vi "TEST Performance Benchmark.vi"() -> ()   [LabVIEW 2011]
panel:
  in  "stop":bool
  in  "source?":bool=TRUE
  in  "Reset Best Time":bool
  out "Best Round Trip Time (ms)":u32
  in  "Parse":bool=TRUE
  in  "Generate":bool=TRUE
  out "Round Trip Time (ms)":u32
  out "Data Round Trip Success?":bool
  in  "Cluster":T1={"Array"=[{"Array"=[{"Array"=[{"Boolean"=FALSE, "Numeric"=0.0, "Numeric 2"=0.0, "Numeric 3"=0.0, "Numeric 4"=0.0}, {"Boolean"=FALSE, "Numeric"=0.0, "Numeric 2"=0.0, "Numeric 3"=0.0, "Numeric 4"=0.0}, {"Boolean"=FALSE, "Numeric"=0.0, "Numeric 2"=0.0, "Numeric 3"=0.0, "Numeric 4"=1.0}], "Numeric"=0.0, "Numeric 2"=0.0, "Numeric 3"=0.0, "Numeric 4"=0.0}, {"Array"=[{"Boolean"=FALSE, "Numeric"=0.0, "Numeric 2"=0.0, "Numeric 3"=0.0, "Numeric 4"=0.0}, {"Boolean"=FALSE, "Numeric"=0.0, "Numeric 2"=0.0, "Numeric 3"=0.0, "Numeric 4"=0.0}, {"Boolean"=FALSE, "Numeric"=0.0, "Numeric 2"=1.0, "Numeric 3"=0.0, "Numeric 4"=0.0}], "Numeric"=0.0, "Numeric 2"=0.0, "Numeric 3"=0.0, "Numeric 4"=0.0}, {"Array"=[{"Boolean"=FALSE, "Numeric"=0.0, "Numeric 2"=0.0, "Numeric 3"=0.0, "Numeric 4"=1.0}, {"Boolean"=FALSE, "Numeric"=0.0, "Numeric 2"=0.0, "Numeric 3"=0.0, "Numeric 4"=0.0}, {"Boolean"=FALSE, "Numeric"=0.0, "Numeric 2"=0.0, "Numeric 3"=0.0, "Numeric 4"=1.0}], "Numeric"=0.0, "Numeric 2"=0.0, "Numeric 3"=0.0, "Numeric 4"=0.0}], "Cluster 2"={"Boolean"=FALSE, "Numeric"=0.0, "Numeric 2"=0.0, "Numeric 3"=0.0, "Numeric 4"=0.0}}, {"Array"=[], "Cluster 2"={"Boolean"=FALSE, "Numeric"=0.0, "Numeric 2"=0.0, "Numeric 3"=0.0, "Numeric 4"=0.0}}, {"Array"=[], "Cluster 2"={"Boolean"=FALSE, "Numeric"=0.0, "Numeric 2"=0.0, "Numeric 3"=0.0, "Numeric 4"=0.0}}, {"Array"=[{"Array"=[{"Boolean"=FALSE, "Numeric"=0.0, "Numeric 2"=0.0, "Numeric 3"=0.0, "Numeric 4"=0.0}, {"Boolean"=FALSE, "Numeric"=0.0, "Numeric 2"=0.0, "Numeric 3"=0.0, "Numeric 4"=0.0}, {"Boolean"=FALSE, "Numeric"=0.0, "Numeric 2"=0.0, "Numeric 3"=0.0, "Numeric 4"=1.0}], "Numeric"=0.0, "Numeric 2"=0.0, "Numeric 3"=0.0, "Numeric 4"=0.0}, {"Array"=[{"Boolean"=FALSE, "Numeric"=0.0, "Numeric 2"=0.0, "Numeric 3"=0.0, "Numeric 4"=0.0}, {"Boolean"=FALSE, "Numeric"=0.0, "Numeric 2"=0.0, "Numeric 3"=0.0, "Numeric 4"=0.0}, {"Boolean"=FALSE, "Numeric"=0.0, "Numeric 2"=0.0, "Numeric 3"=0.0, "Numeric 4"=1.0}], "Numeric"=0.0, "Numeric 2"=0.0, "Numeric 3"=0.0, "Numeric 4"=0.0}, {"Array"=[{"Boolean"=FALSE, "Numeric"=0.0, "Numeric 2"=0.0, "Numeric 3"=0.0, "Numeric 4"=0.0}, {"Boolean"=FALSE, "Numeric"=0.0, "Numeric 2"=0.0, "Numeric 3"=0.0, "Numeric 4"=0.0}, {"Boolean"=FALSE, "Numeric"=0.0, "Numeric 2"=0.0, "Numeric 3"=0.0, "Numeric 4"=1.0}], "Numeric"=0.0, "Numeric 2"=0.0, "Numeric 3"=0.0, "Numeric 4"=1.0}], "Cluster 2"={"Boolean"=FALSE, "Numeric"=0.0, "Numeric 2"=0.0, "Numeric 3"=0.0, "Numeric 4"=0.0}}], "Cluster 2"={"Boolean"=FALSE, "Numeric"=0.0, "Numeric 2"=0.0, "Numeric 3"=0.0, "Numeric 4"=0.0}, "Cluster 3"={"Boolean"=FALSE, "Numeric"=0.0, "Numeric 2"=0.0, "Numeric 3"=0.0, "Numeric 4"=0.0}, "Cluster 4"={"Boolean"=TRUE, "Numeric"=0.0, "Numeric 2"=0.0, "Numeric 3"=0.0, "Numeric 4"=0.0}, "Cluster 5"={"Boolean"=TRUE, "Numeric"=0.0, "Numeric 2"=0.0, "Numeric 3"=0.0, "Numeric 4"=0.0}, "Array 2"=[{"Array"=[{"Array"=[{"Boolean"=FALSE, "Numeric"=0.0, "Numeric 2"=0.0, "Numeric 3"=0.0, "Numeric 4"=0.0}, {"Boolean"=FALSE, "Numeric"=0.0, "Numeric 2"=0.0, "Numeric 3"=0.0, "Numeric 4"=0.0}, {"Boolean"=FALSE, "Numeric"=0.0, "Numeric 2"=0.0, "Numeric 3"=0.0, "Numeric 4"=1.0}], "Numeric"=0.0, "Numeric 2"=0.0, "Numeric 3"=0.0, "Numeric 4"=0.0}, {"Array"=[{"Boolean"=FALSE, "Numeric"=0.0, "Numeric 2"=0.0, "Numeric 3"=0.0, "Numeric 4"=0.0}, {"Boolean"=FALSE, "Numeric"=0.0, "Numeric 2"=0.0, "Numeric 3"=0.0, "Numeric 4"=0.0}, {"Boolean"=FALSE, "Numeric"=0.0, "Numeric 2"=1.0, "Numeric 3"=0.0, "Numeric 4"=0.0}], "Numeric"=0.0, "Numeric 2"=0.0, "Numeric 3"=0.0, "Numeric 4"=0.0}, {"Array"=[{"Boolean"=FALSE, "Numeric"=0.0, "Numeric 2"=0.0, "Numeric 3"=0.0, "Numeric 4"=1.0}, {"Boolean"=FALSE, "Numeric"=0.0, "Numeric 2"=0.0, "Numeric 3"=0.0, "Numeric 4"=0.0}, {"Boolean"=FALSE, "Numeric"=0.0, "Numeric 2"=0.0, "Numeric 3"=0.0, "Numeric 4"=1.0}], "Numeric"=0.0, "Numeric 2"=0.0, "Numeric 3"=0.0, "Numeric 4"=0.0}], "Cluster 2"={"Boolean"=FALSE, "Numeric"=0.0, "Numeric 2"=0.0, "Numeric 3"=0.0, "Numeric 4"=0.0}}, {"Array"=[], "Cluster 2"={"Boolean"=FALSE, "Numeric"=0.0, "Numeric 2"=0.0, "Numeric 3"=0.0, "Numeric 4"=0.0}}, {"Array"=[], "Cluster 2"={"Boolean"=FALSE, "Numeric"=0.0, "Numeric 2"=0.0, "Numeric 3"=0.0, "Numeric 4"=0.0}}, {"Array"=[{"Array"=[{"Boolean"=FALSE, "Numeric"=0.0, "Numeric 2"=0.0, "Numeric 3"=0.0, "Numeric 4"=0.0}, {"Boolean"=FALSE, "Numeric"=0.0, "Numeric 2"=0.0, "Numeric 3"=0.0, "Numeric 4"=0.0}, {"Boolean"=FALSE, "Numeric"=0.0, "Numeric 2"=0.0, "Numeric 3"=0.0, "Numeric 4"=1.0}], "Numeric"=0.0, "Numeric 2"=0.0, "Numeric 3"=0.0, "Numeric 4"=0.0}, {"Array"=[{"Boolean"=FALSE, "Numeric"=0.0, "Numeric 2"=0.0, "Numeric 3"=0.0, "Numeric 4"=0.0}, {"Boolean"=FALSE, "Numeric"=0.0, "Numeric 2"=0.0, "Numeric 3"=0.0, "Numeric 4"=0.0}, {"Boolean"=FALSE, "Numeric"=0.0, "Numeric 2"=0.0, "Numeric 3"=0.0, "Numeric 4"=1.0}], "Numeric"=0.0, "Numeric 2"=0.0, "Numeric 3"=0.0, "Numeric 4"=0.0}, {"Array"=[{"Boolean"=FALSE, "Numeric"=0.0, "Numeric 2"=0.0, "Numeric 3"=0.0, "Numeric 4"=0.0}, {"Boolean"=FALSE, "Numeric"=0.0, "Numeric 2"=0.0, "Numeric 3"=0.0, "Numeric 4"=0.0}, {"Boolean"=FALSE, "Numeric"=0.0, "Numeric 2"=0.0, "Numeric 3"=0.0, "Numeric 4"=1.0}], "Numeric"=0.0, "Numeric 2"=0.0, "Numeric 3"=0.0, "Numeric 4"=1.0}], "Cluster 2"={"Boolean"=FALSE, "Numeric"=0.0, "Numeric 2"=0.0, "Numeric 3"=0.0, "Numeric 4"=0.0}}]}
  # "261"
  # "231 - 2.0.4 source"
  # "225 - 2.0.4 built"
  # "233 - 2.0.3 built"
  # "235 - 2.0.2a01 built"
  # "548 - 2.0 built"
  # "948 - 1.0 built"
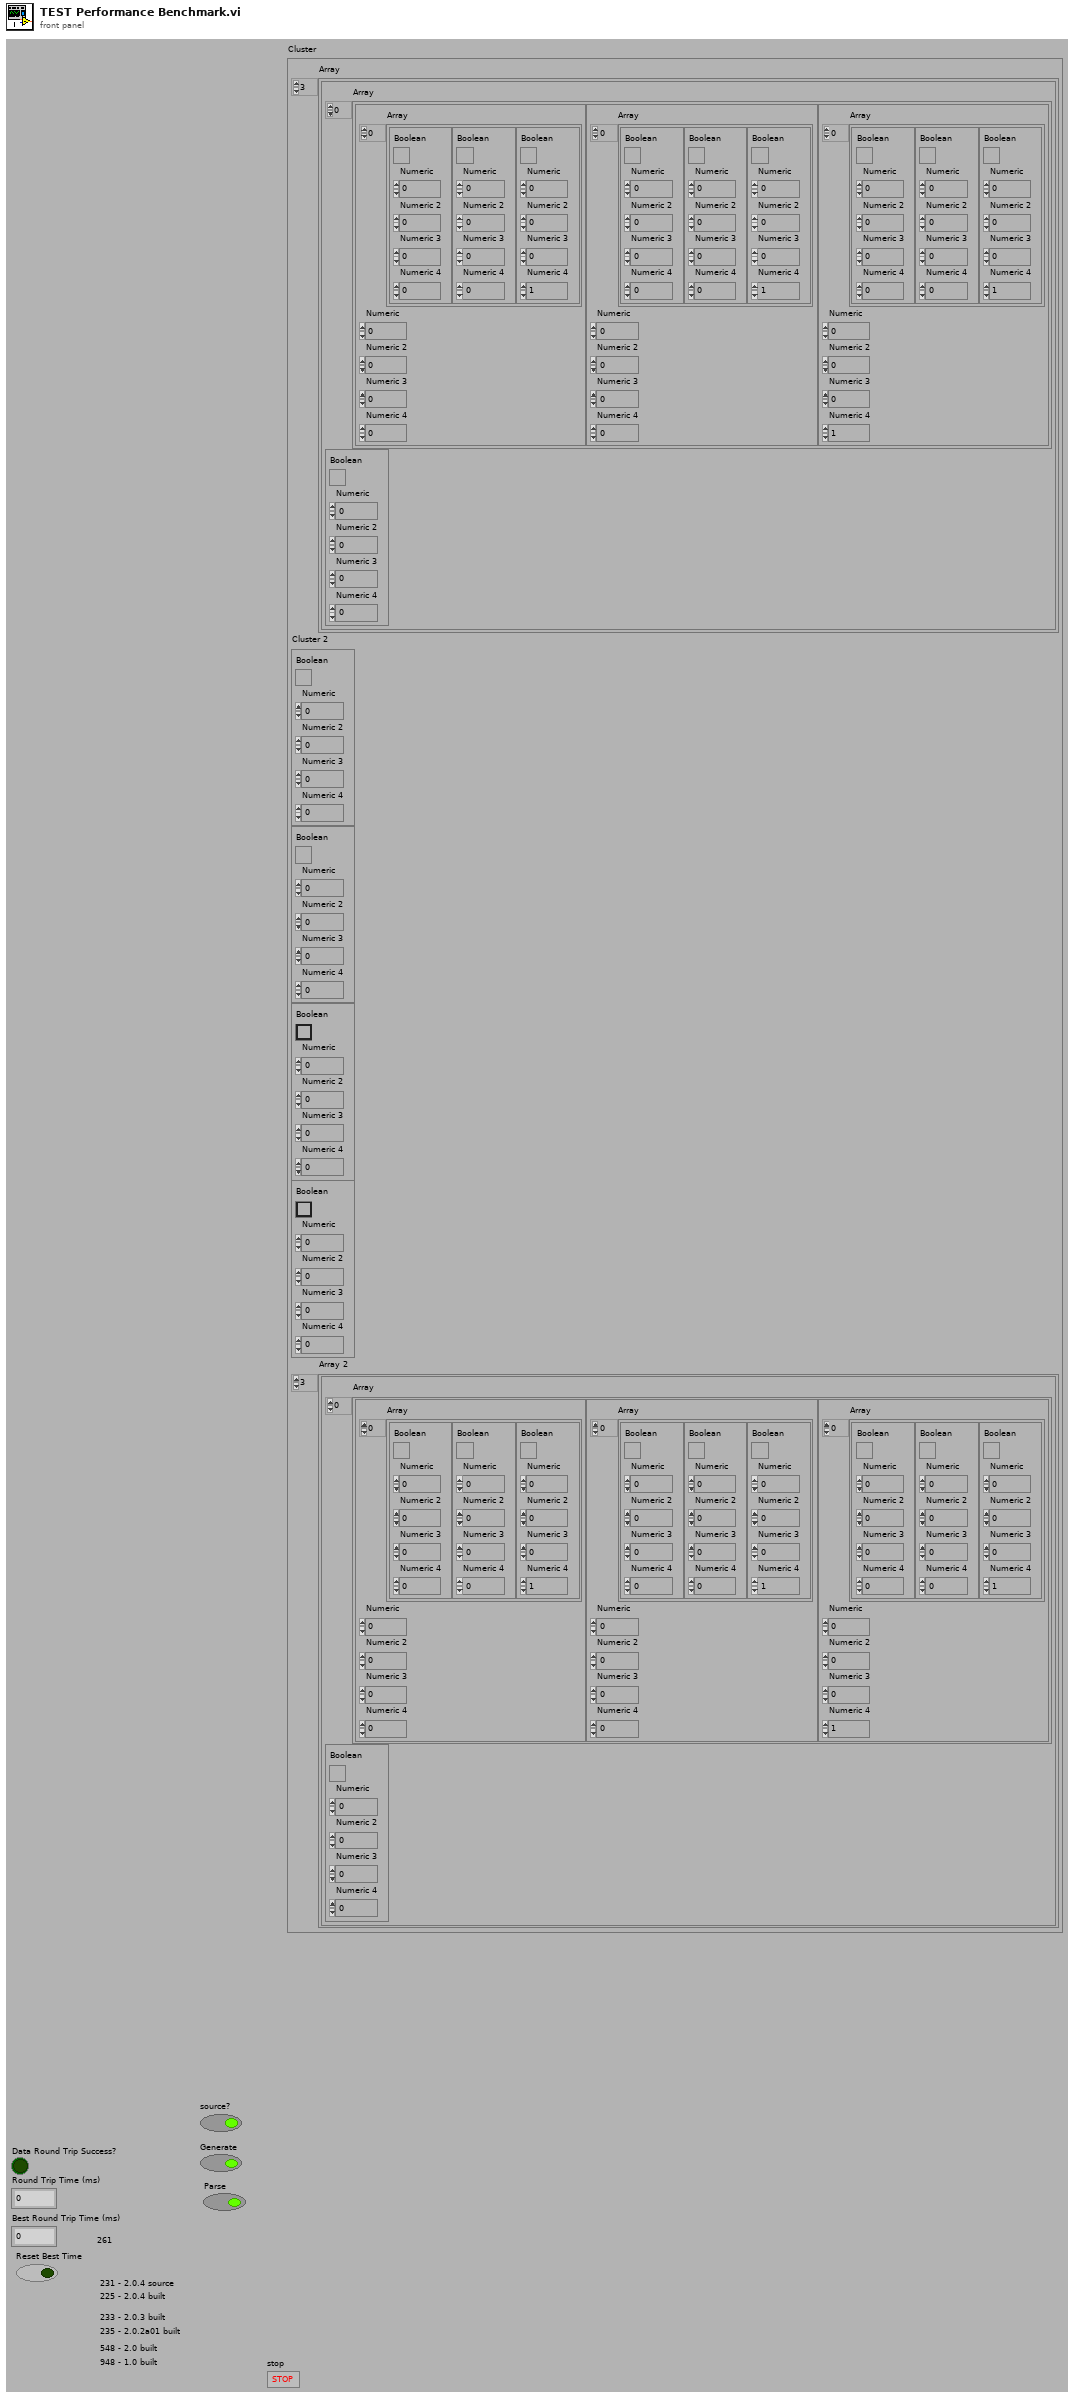
[diagram p1: front panel]
types:
  T1 = cluster{"Array":cluster{"Array":cluster{"Array":cluster{"Boolean":bool, "Numeric":dbl, "Numeric 2":dbl, "Numeric 3":dbl, "Numeric 4":dbl}[], "Numeric":dbl, "Numeric 2":dbl, "Numeric 3":dbl, "Numeric 4":dbl}[], "Cluster 2":cluster{"Boolean":bool, "Numeric":dbl, "Numeric 2":dbl, "Numeric 3":dbl, "Numeric 4":dbl}}[], "Cluster 2":cluster{"Boolean":bool, "Numeric":dbl, "Numeric 2":dbl, "Numeric 3":dbl, "Numeric 4":dbl}, "Cluster 3":cluster{"Boolean":bool, "Numeric":dbl, "Numeric 2":dbl, "Numeric 3":dbl, "Numeric 4":dbl}, "Cluster 4":cluster{"Boolean":bool, "Numeric":dbl, "Numeric 2":dbl, "Numeric 3":dbl, "Numeric 4":dbl}, "Cluster 5":cluster{"Boolean":bool, "Numeric":dbl, "Numeric 2":dbl, "Numeric 3":dbl, "Numeric 4":dbl}, "Array 2":cluster{"Array":cluster{"Array":cluster{"Boolean":bool, "Numeric":dbl, "Numeric 2":dbl, "Numeric 3":dbl, "Numeric 4":dbl}[], "Numeric":dbl, "Numeric 2":dbl, "Numeric 3":dbl, "Numeric 4":dbl}[], "Cluster 2":cluster{"Boolean":bool, "Numeric":dbl, "Numeric 2":dbl, "Numeric 3":dbl, "Numeric 4":dbl}}[]}
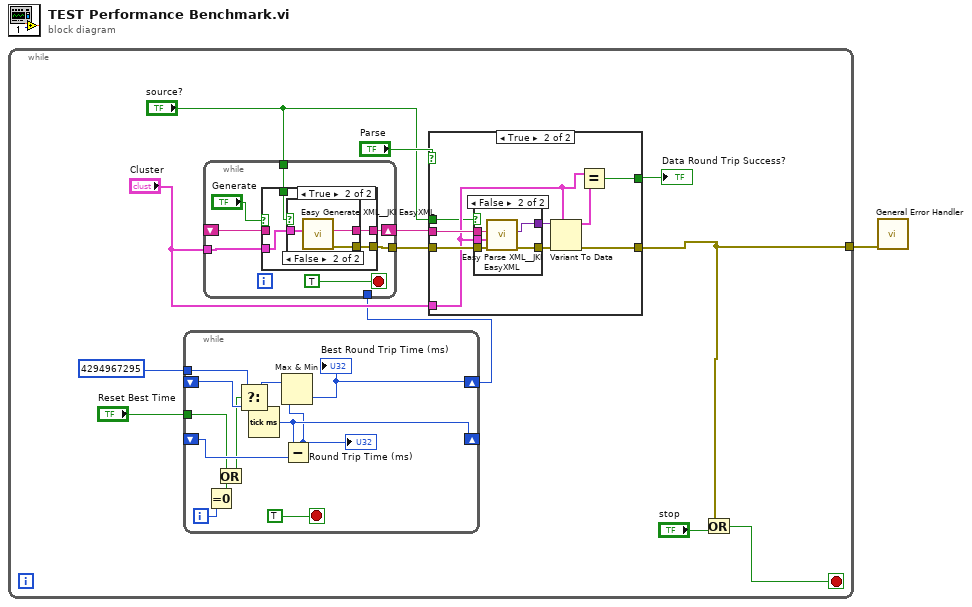
[diagram p0: block diagram]
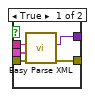
[diagram p3: hidden frame]
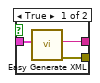
[diagram p5: hidden frame]
diagram:
  n1 = while {
    tunnel: [w2] -> w1
    stop <- w3 stop-if-true
    n2 = while {
      shift-right: [w63] -> _
      shift-left: _ -> [w56]
      shift-right: [w61] -> w6
      shift-left: _ -> [w59]
      tunnel: u32 4294967295 -> [w57]
      tunnel: "Reset Best Time" -> [w53]
      i -> [w55]
      stop <- TRUE stop-if-true
      n3 = Equal To 0?(x=w55) -> (x = 0?=w54:bool)
      n4 = Or(x=w53, y=w54) -> (x .or. y?=w52:bool)
      n5 = Select(t=w57, s=w52, f=w59) -> (s? t:f=w58:u32)
      n6 = Tick Count (ms)() -> (millisecond timer value=w63:u32)
      n7 = Subtract(x=w63, y=w56) -> (x-y=w60:u32)
      "Round Trip Time (ms)" <- w60
      n8 = Max & Min(x=w58, y=w60) -> (min(x,y)=w61:u32)  [unwired: 1 out]
      "Best Round Trip Time (ms)" <- w61
    }
    n9 = while {
      tunnel: [w39] -> w12
      tunnel: "Cluster" -> [w38]
      shift-right: [w40] -> w13
      shift-left: _ -> [w36]
      tunnel: w6 -> [_]
      tunnel: "source?" -> [w34]
      stop <- TRUE stop-if-true
      n10 = case shown="True" "Generate" {
        tunnel: [w41 w45] -> w40
        tunnel: [_ w44] -> w39
        tunnel: w38 -> [_ w43]
        tunnel: w36 -> [w41 _]
        tunnel: w34 -> [_ w42]
        frame False {
        }
        frame True {
          n11 = case shown="False" w42 {
            tunnel: [w48 w51] -> w45
            tunnel: [w47 w50] -> w44
            tunnel: w43 -> [w46 w49]
            frame True {
              n12 = call "Easy Generate XML.vi"("LabVIEW Data"=w46) -> ("error out"=w47:errorcluster, "XML String"=w48:string)  [unwired: 9 in]
            }
            frame False {
              n13 = call <vilib>:"Easy Generate XML__JKI EasyXML.vi"("LabVIEW Data"=w49) -> ("error out"=w50:errorcluster, "XML String"=w51:string)  [unwired: 9 in]
            }
          }
        }
      }
    }
    n14 = case shown="True" "Parse" {
      tunnel: w13 -> [_ w23]
      tunnel: w12 -> [w14 w22]
      tunnel: [w14 w19] -> w2
      tunnel: "Cluster" -> [_ w18]
      tunnel: [_ w16] -> w10
      tunnel: "source?" -> [_ w15]
      frame False {
      }
      frame True {
        n15 = case shown="False" w15 {
          tunnel: w23 -> [w28 w33]
          tunnel: w22 -> [w27 w32]
          tunnel: [w26 w31] -> w21
          tunnel: [w25 w30] -> w20
          tunnel: w18 -> [w24 w29]
          frame True {
            n16 = call "Easy Parse XML.vi"("error in (no error)"=w27, "LabVIEW Data (Type)"=w24, "XML String"=w28) -> ("error out"=w25:errorcluster, "LabVIEW Data"=w26:variant)  [unwired: 7 in]
          }
          frame False {
            n17 = call <vilib>:"Easy Parse XML__JKI EasyXML.vi"("error in (no error)"=w32, "LabVIEW Data (Type)"=w29, "XML String"=w33) -> ("error out"=w30:errorcluster, "LabVIEW Data"=w31:variant)  [unwired: 7 in]
          }
        }
        n18 = Variant To Data(error in=w20, type=w18, Variant=w21) -> (data=w17:T1, error out=w19:errorcluster)
        n19 = Equal?(x=w18, y=w17) -> (x = y?=w16:bool)
      }
    }
    "Data Round Trip Success?" <- w10
    n20 = Or(x=w2, y="stop") -> (x .or. y?=w3:bool)
  }
  n21 = call <vilib>:"General Error Handler.vi"("error in (no error)"=w1) -> ()  [unwired: 10 in, 5 out]
